vi "Breaker Safety.vi"(0 "Breakers":bool[](array[boolean]), 1 "Timeout (ms)":u32=60000, 2 "Pop Count":u8=2) -> (3 "Halt":bool, 4 "Warning":bool, 5 "Cooldown":dbl, 6 "Remaining":u8)   [LabVIEW 2015]
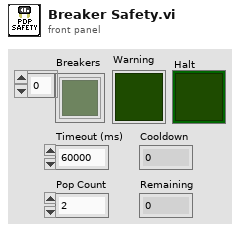
[diagram p1: front panel]
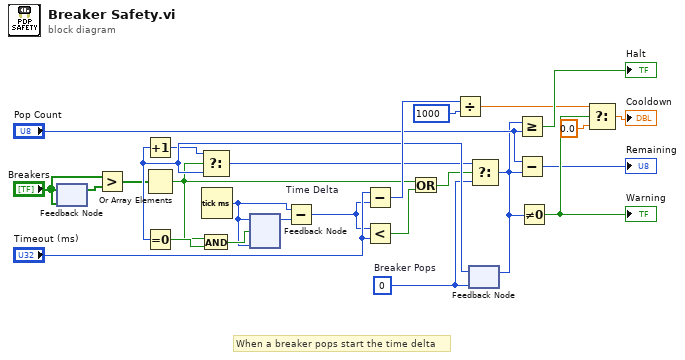
[diagram p0: block diagram]
diagram:
  w11 = u8 0  # Breaker Pops
  # "When a breaker pops start the time delta"
  n1 = feedback #1("Breakers") -> (w15:bool[])
  n2 = feedback-in #1("Breakers") -> ()
  n3 = Greater?(x="Breakers", y=w15) -> (0:w16:bool[])
  n4 = Or Array Elements(Boolean array=w16) -> (logical OR=w4:bool)
  n5 = Tick Count (ms)() -> (millisecond timer value=w10:u32)
  n6 = feedback #2(w10) -> (w9:u32)
  n7 = Subtract "Time Delta"(x=w10, y=w9) -> (x-y=w6:u32)
  n8 = Subtract(x="Timeout (ms)", y=w6) -> (x-y=w20:u32)
  n9 = Less?(x=w6, y="Timeout (ms)") -> (x < y?=w19:bool)
  n10 = Or(x=w4, y=w19) -> (x .or. y?=w5:bool)
  n11 = Divide(x=w20, y=u32 1000) -> (x/y=w7:dbl)
  n12 = feedback #3(w11) -> (w18:u8)
  n13 = Increment(x=w18) -> (x+1=w12:u8)
  n14 = Equal To 0?(x=w18) -> (x = 0?=w17:bool)
  n15 = Select(t=w12, s=w4, f=w18) -> (s? t:f=w13:u8)
  n16 = And(x=w4, y=w17) -> (x .and. y?=w14:bool)
  n17 = feedback-in #2(w10, w14) -> ()
  n18 = Select(t=w13, s=w5, f=w11) -> (s? t:f=w2:u8)
  n19 = feedback-in #3(w2) -> ()
  n20 = Greater Or Equal?(x=w2, y="Pop Count") -> (x >= y?=→"Halt":bool)
  n21 = Subtract(x="Pop Count", y=w2) -> (x-y=→"Remaining":u8)
  n22 = Not Equal To 0?(x=w2) -> (x != 0?=w24:bool)
  "Warning" <- w24
  n23 = Select(t=w7, s=w24, f=0.0) -> (s? t:f=→"Cooldown":dbl)
